vi "RubikOpGroup.vi"(2 "error in":errorcluster, 3 "Array of Operations":T2[](array[typedef])) -> (0 "error out":errorcluster)   [LabVIEW 2017]
uses:
  Projekt-RubikLibrary/RubikOps.ctl
  Projekt-RubikLibrary/ServoAbsAngleControl.ctl
  Projekt-RubikLibrary/ServoEnumControl.ctl
  179a9055-43a9-4ddd-994f-a0e33df00949.vi
  3ffa1dd7-a0aa-4dc6-83d2-f4eb2941c70e.vi
  Projekt-RubikLibrary/RubikLibraryRT.lvlib
  Projekt-RubikLibrary/RubikLibrary.lvlib
panel:
  out "Which Op?":enum16{"Servo", "SyncTurn", "Grip"}(ring)
  out "# op":i32
  out "N# Servo":i32
  out "NoWait Servo":bool
  out "Servo Angles":T1
  out "N# Grip":i32
  out "NoWait Grip":bool
  out "Grip":bool
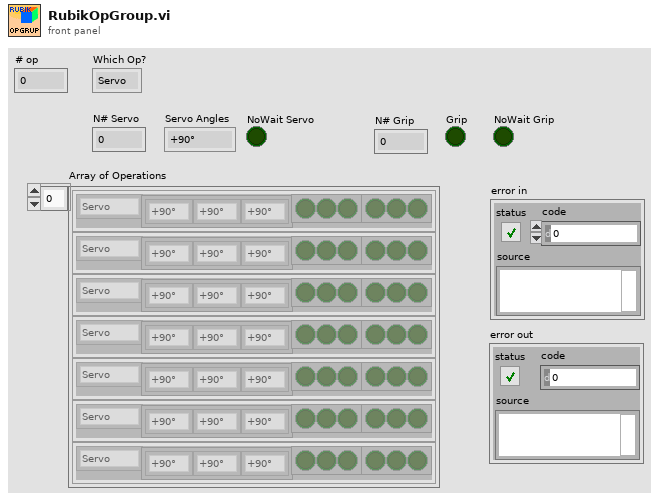
[diagram p1: front panel]
types:
  T1 = typedef "RubikLibrary.lvlib/ServoAbsAngleControl.ctl" = enum16{"+90°", "0°", "-90°"}
  T2 = typedef "RubikLibrary.lvlib/RubikOps.ctl" = cluster{"Device":enum16{"Servo", "SyncTurn", "Grip"}, "Angles":T1[], "Grips":bool[], "NoWaits":bool[]}
  T3 = typedef "RubikLibrary.lvlib/ServoEnumControl.ctl" = enum16{"Left Servo", "Front Servo", "Right Servo"}
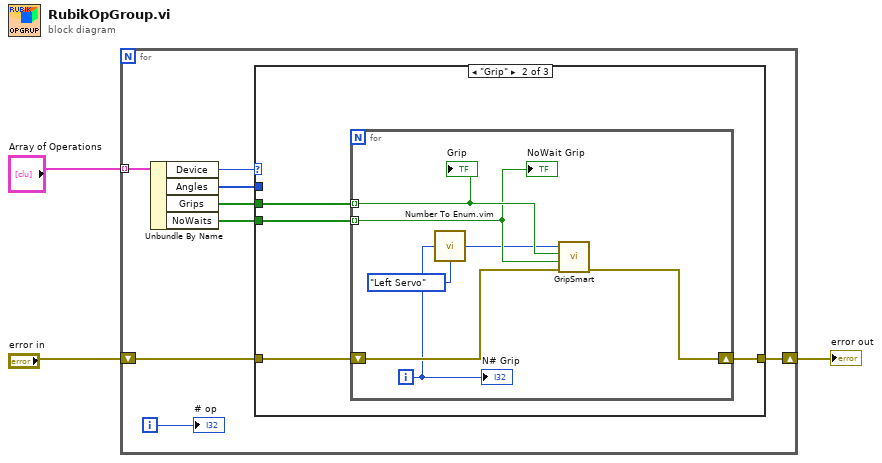
[diagram p0: block diagram]
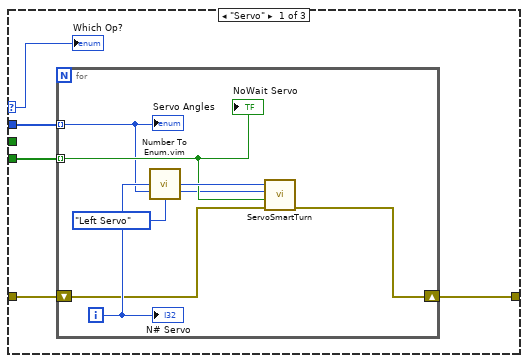
[diagram p2: hidden frame]
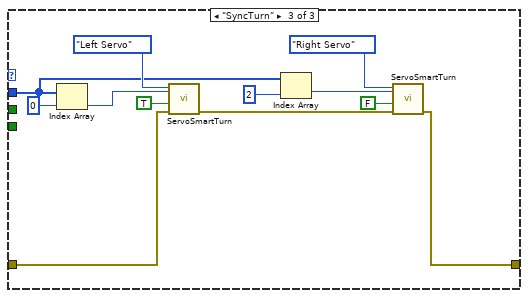
[diagram p3: hidden frame]
diagram:
  n1 = for {
    tunnel: "Array of Operations" -> [w11] mode=indexing
    shift-right: [w5] -> w2
    shift-left: "error in" -> [w6]
    i -> [w4]
    n2 = Unbundle By Name(w11) -> ("Device"=w10:enum16{"Servo", "SyncTurn", "Grip"}, "Angles"=w9:T1[], "Grips"=w8:bool[], "NoWaits"=w7:bool[])
    n3 = case shown="\"Grip\"" w10 {
      selector: w10 -> [w12 _ _]
      tunnel: w9 -> [w16 _ w38]
      tunnel: w8 -> [_ w24 _]
      tunnel: w7 -> [w15 w27 _]
      tunnel: w6 -> [w14 w26 w36]
      tunnel: [w13 w25 w35] -> w5
      frame "Servo" {
        n4 = for {
          tunnel: w16 -> [w17] mode=indexing
          tunnel: w15 -> [w18] mode=indexing
          shift-right: [w19] -> w13
          shift-left: w14 -> [w20]
          i -> [w22]
          n5 = call "Number To Enum.vim"("number"=w22, "enum type"=ServoEnumControl."Left Servo" ("Servo Enum")) -> ("number as enum"=w21:T3)
          n6 = call "ServoSmartTurn.vi"("error in"=w20, "NoWait"=w18, "Turn to (in)"=w17, "Servo"=w21) -> ("error out"=w19:errorcluster)  [unwired: 6 in, 1 out]
          "Servo Angles" <- w17
          "NoWait Servo" <- w18
          "N# Servo" <- w22
        }
        "Which Op?" <- w12
      }
      frame "Grip" {
        n7 = for {
          tunnel: w24 -> [w32] mode=indexing
          tunnel: w27 -> [w31] mode=indexing
          shift-right: [w33] -> w25
          shift-left: w26 -> [w34]
          i -> [w30]
          n8 = call "Number To Enum.vim"("number"=w30, "enum type"=ServoEnumControl."Left Servo" ("Servo Enum")) -> ("number as enum"=w28:T3)
          n9 = call "GripSmart.vi"("error in"=w34, "NoWait"=w31, "Grip closed (in)"=w32, "Servo"=w28) -> ("error out"=w33:errorcluster)  [unwired: 6 in, 1 out]
          "Grip" <- w32
          "NoWait Grip" <- w31
          "N# Grip" <- w30
        }
      }
      frame "SyncTurn" {
        n10 = Index Array(array=w38, index=0) -> (element=w41:T1)
        n11 = call "ServoSmartTurn.vi"("error in"=w36, "NoWait"=TRUE, "Turn to (in)"=w41, "Servo"=ServoEnumControl."Left Servo") -> ("error out"=w40:errorcluster)  [unwired: 6 in, 1 out]
        n12 = Index Array(array=w38, index=2) -> (element=w37:T1)
        n13 = call "ServoSmartTurn.vi"("error in"=w40, "NoWait"=FALSE, "Turn to (in)"=w37, "Servo"=ServoEnumControl."Right Servo") -> ("error out"=w35:errorcluster)  [unwired: 6 in, 1 out]
      }
    }
    "# op" <- w4
  }
  "error out" <- w2
